vi "EMD8216 port read.vi"(10 "port":u8, 11 "CardID":u32) -> (1 "data":u8, 3 "error_code":u32)   [LabVIEW 2015, in "EMD8216_64.lvlib"]
doc: "EMD8216Status EMD8216_port_read(u32 CardID,u8 port,u8 *data);"
uses:
  EMD8216_64.lvlib
  EMD8216_64.dll
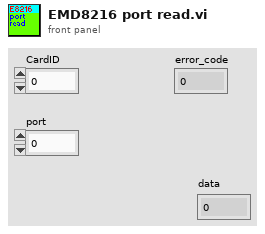
[diagram p1: front panel]
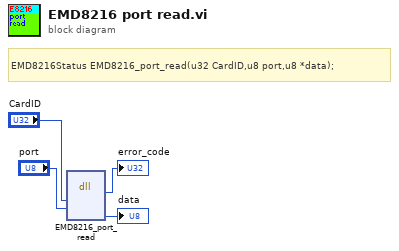
[diagram p0: block diagram]
diagram:
  # "EMD8216Status EMD8216_port_read(u32 CardID,u8 port,u8 *data);"
  n1 = dll-call lib="C:/Users/jeff.lin.MINAIK/Documents/Soulkai/Labview/io/EMD8216_64/EMD8216_64/EMD8216_64.*" fn="EMD8216_port_read"("CardID"="CardID", "port"="port") -> ("return type"=→"error_code":u32, "data"=→"data":u8)  [unwired: 6 in, 2 out]
